vi "DivideByZero.vi"() -> ()   [LabVIEW 2015]
panel:
  out "Boolean":bool
  out "Numeric 3":dbl
  in  "Numeric 2":dbl
  in  "Numeric":dbl
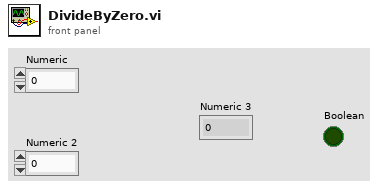
[diagram p1: front panel]
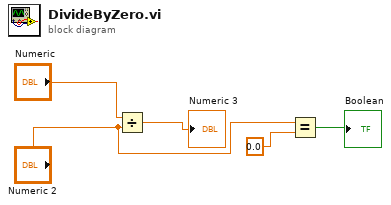
[diagram p0: block diagram]
diagram:
  n1 = Divide(x="Numeric", y="Numeric 2") -> (x/y=→"Numeric 3":dbl)
  n2 = Equal?(x="Numeric 2", y=0.0 ("Numeric 4")) -> (x = y?=→"Boolean":bool)
